vi "http handle header.vi"(9 "header field data":string, 10 "header field name":string, 11 "application request in":T1) -> (3 "application request out":T1)   [LabVIEW 2013]
uses:
  http request.ctl
  http method.ctl
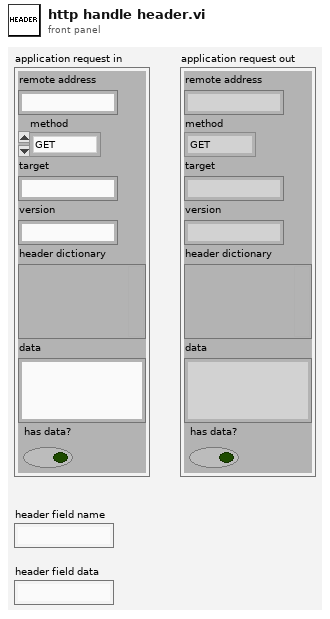
[diagram p1: front panel]
types:
  T1 = typedef "http request.ctl" = cluster{"remote address":string, "method":T2, "target":string, "version":string, "header dictionary":variant, "data":string, "has data?":bool}
  T2 = typedef "http method.ctl" = enum16{"GET", "POST", "PUT", "DELETE", "HEAD", "OPTIONS", "upgrade"}
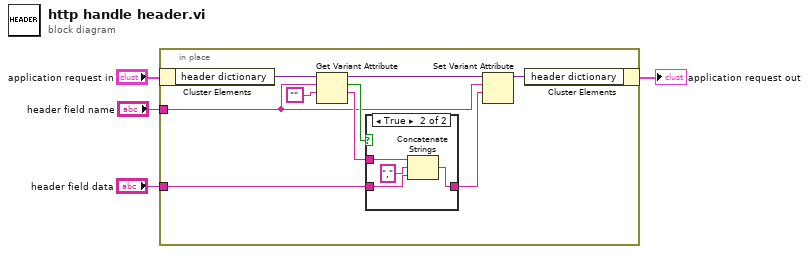
[diagram p0: block diagram]
diagram:
  n1 = in-place {
    in-place-border: "header field name" -> [w5]
    in-place-border: "header field data" -> [w8]
    n2 = in-place-cluster #1("application request in") -> ("header dictionary"=w12:variant)
    n3 = Get Variant Attribute(Variant=w12, name=w5, default value (empty Variant)="") -> (duplicate Variant=w11:variant, found=w9:bool, value=w7:string)  [unwired: 1 in, 1 out]
    n4 = case shown="True" w9 {
      tunnel: w8 -> [w14 w18]
      tunnel: w7 -> [_ w17]
      tunnel: [w14 w15] -> w6
      frame False {
      }
      frame True {
        n5 = Concatenate Strings(w17, "," ("string"), w18) -> (w15:string)
      }
    }
    n6 = Set Variant Attribute(Variant=w11, name=w5, value=w6) -> (Variant out=w13:variant)  [unwired: 1 in, 2 out]
    n7 = in-place-cluster #1("header dictionary"=w13) -> (→"application request out":T1)
  }
